vi "End Game.vi"(11 "Team in":refnum<class "Team.lvclass">) -> (3 "Team out":refnum<class "Team.lvclass">)   [LabVIEW 2020, in "SquareBattle.lvlib" / "Team.lvclass"]
uses:
  Team.lvclass
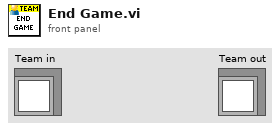
[diagram p1: front panel]
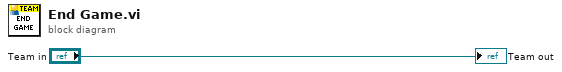
[diagram p0: block diagram]
diagram:
  "Team out" <- "Team in"
